vi "S2DS_Add user.vi"(8 "error in (no error)":errorcluster, 11 "new user":string) -> (0 "error out":errorcluster)   [LabVIEW 2025]
uses:
  <vilib>/Utility/config.llb/Read Key (I32).vi
  <vilib>/Utility/config.llb/Write Key (I32).vi
  <vilib>/Utility/config.llb/Write Key (String).vi
  <vilib>/Utility/config.llb/NI_LVConfig.lvlib
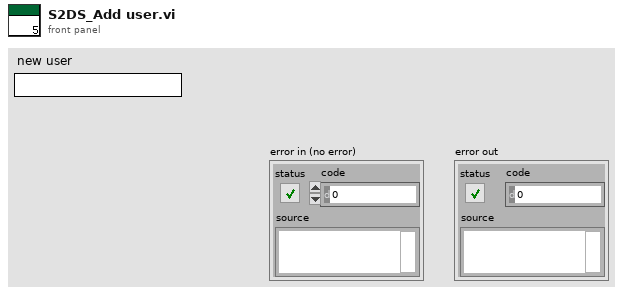
[diagram p1: front panel]
types:
  T1 = typedef "NI_LVConfig.lvlib/Config Data RefNum.ctl" = refnum<k1>
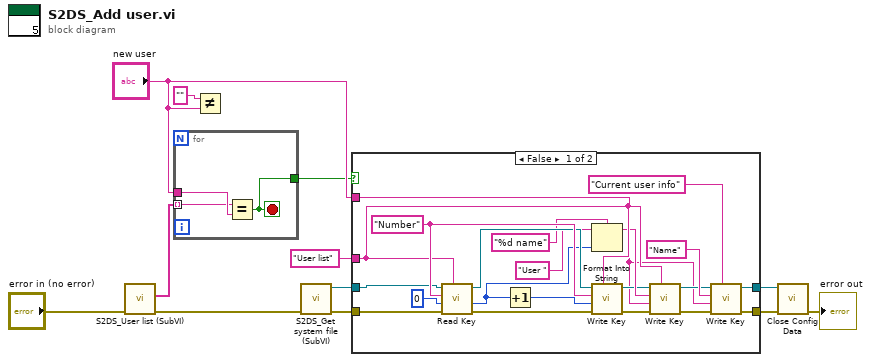
[diagram p0: block diagram]
diagram:
  n1 = call "S2DS_User list (SubVI).vi"("error in (no error)"="error in (no error)") -> ("error out"=w4:errorcluster, "User list"=w3:string[])  [unwired: 7 in, 2 out]
  n2 = for {
    tunnel: w3 -> [w14] mode=indexing
    tunnel: "new user" -> [w15]
    tunnel: [w13] -> w1
    stop <- w13 stop-if-true
    n3 = Equal?(x=w14, y=w15) -> (x = y?=w13:bool)
  }
  n4 = Not Equal?(x="", y="new user") -> ()  [unwired: 1 out]
  n5 = call "S2DS_Get system file (SubVI).vi"("error in (no error)"=w4) -> ("error out"=w9:errorcluster, "Refnum out"=w10:T1)  [unwired: 9 in]
  n6 = case shown="False" w1 {
    tunnel: [w16 w37] -> w7
    tunnel: [w17 w38] -> w8
    tunnel: w9 -> [w33 w37]
    tunnel: w10 -> [w34 w38]
    tunnel: "new user" -> [w19 _]
    tunnel: "User list" ("section") -> [w29 _]
    frame False {
      w35 = "Number" ("key")
      n7 = call-poly <vilib>:"Read Key.vi"("section"=w29, "error in (no error)"=w33, "default value"=0, "key"=w35, "refnum"=w34) -> ("error out"=w32:errorcluster, "value"=w26:i32, "refnum out"=w31:T1)  [unwired: 3 in, 1 out]
      n8 = Increment(x=w26) -> (x+1=w30:i32)
      n9 = Format Into String(format string="%d name", initial string="User " ("key"), w26) -> (resulting string=w25:string)  [unwired: 1 in, 1 out]
      n10 = call-poly <vilib>:"Write Key.vi"("section"=w29, "error in (no error)"=w32, "value"=w30, "key"=w35, "refnum"=w31) -> ("error out"=w23:errorcluster, "refnum out"=w24:T1)  [unwired: 4 in, 1 out]
      n11 = call-poly <vilib>:"Write Key.vi"("section"=w29, "error in (no error)"=w23, "value"=w19, "key"=w25, "refnum"=w24) -> ("error out"=w18:errorcluster, "refnum out"=w20:T1)  [unwired: 4 in, 1 out]
      n12 = call-poly <vilib>:"Write Key.vi"("section"="Current user info", "error in (no error)"=w18, "value"=w19, "key"="Name", "refnum"=w20) -> ("error out"=w16:errorcluster, "refnum out"=w17:T1)  [unwired: 4 in, 1 out]
    }
    frame True {
    }
  }
  n13 = call <vilib>:"Close Config Data.vi"("error in (no error)"=w7, "refnum"=w8) -> ("error out"=→"error out":errorcluster)  [unwired: 8 in, 1 out]
